vi "Voorbeeld_Event_Driven_Programmeren_01_timing.vi"() -> ()   [LabVIEW 2019]
panel:
  out "Boolean":bool
  in  "stop":bool
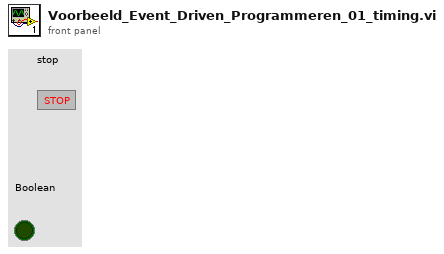
[diagram p1: front panel]
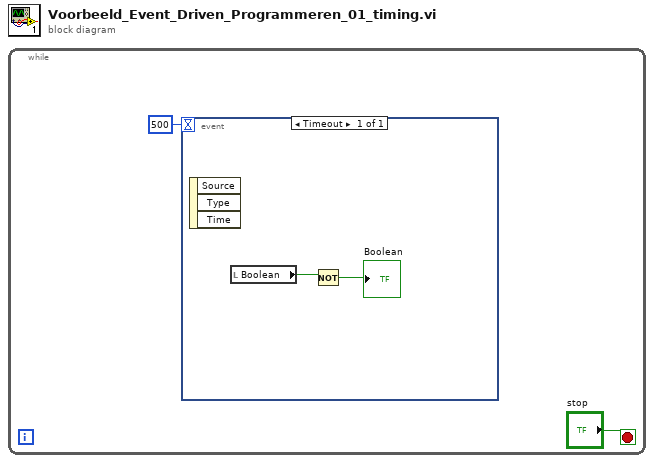
[diagram p0: block diagram]
diagram:
  n1 = while {
    stop <- "stop" stop-if-true
    n2 = event shown="[0] Timeout" {
      selector: _ -> [_]
      dyn-events: _ -> [_]
      timeout: 500 -> [_]
      event Timeout {
        n3 = event-data() -> ()  [unwired: 1 in, 3 out]
        n4 = local read "Boolean"() -> (w4:bool)
        n5 = Not(x=w4) -> (.not. x?=→"Boolean":bool)
      }
    }
  }
